vi "MeasurementServer_AddOCVMeasurementEvent.vi"(11 "gRPCid in":T1) -> (2 "QueryServer_OCVMeasurement":refnum<user-event>, 3 "gRPCid":T1)   [LabVIEW 2019, in "labview-grpc-measurement-server.lvlib"]
uses:
  labview-grpc-measurement-server.lvlib
  MeasurementServer_InvokeEventData.ctl
  MeasurementServer_gRPCid.ctl
  a66ee327-264b-4784-bac1-fff8ba4a2692.vi
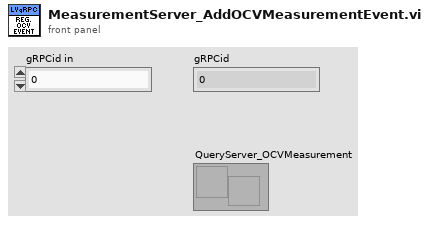
[diagram p1: front panel]
types:
  T1 = typedef "labview-grpc-measurement-server.lvlib/MeasurementServer_gRPCid.ctl" = u64
  T2 = typedef "labview-grpc-measurement-server.lvlib/MeasurementServer_InvokeEventData.ctl" = cluster{"gRPCid":T1}
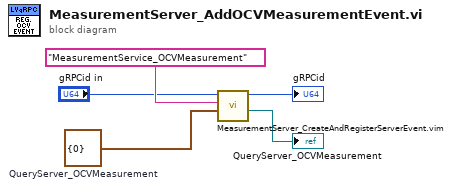
[diagram p0: block diagram]
diagram:
  w1 = T2 {"gRPCid"=0}  # QueryServer_OCVMeasurement
  n1 = call "MeasurementServer_CreateAndRegisterServerEvent.vim"("event in"=w1, "name"="MeasurementService_OCVMeasurement", "gRPCid in"="gRPCid in") -> ("event"=→"QueryServer_OCVMeasurement":refnum<user-event>, "gRPCid"=→"gRPCid":T1)  [unwired: 7 in]
